vi "Add Record.vi"(8 "error in (no error)":errorcluster, 9 "Channel List":string, 10 "Waveforms":T1(array[cluster]), 11 "Live Graph Plotter in":refnum<class "Live Graph Plotter.lvclass">) -> (0 "error out":errorcluster, 3 "Live Graph Plotter out":refnum<class "Live Graph Plotter.lvclass">)   [LabVIEW 2025, in "Live Graph Plotter.lvclass"]
uses:
  Live Graph Plotter.lvclass
  Live Graph Plotter.lvclass/Live Graph Plotter.ctl
  <vilib>/ErrorRing/Error Ring.xnode
  <vilib>/Utility/error.llb/Error Cluster From Error Code.vi
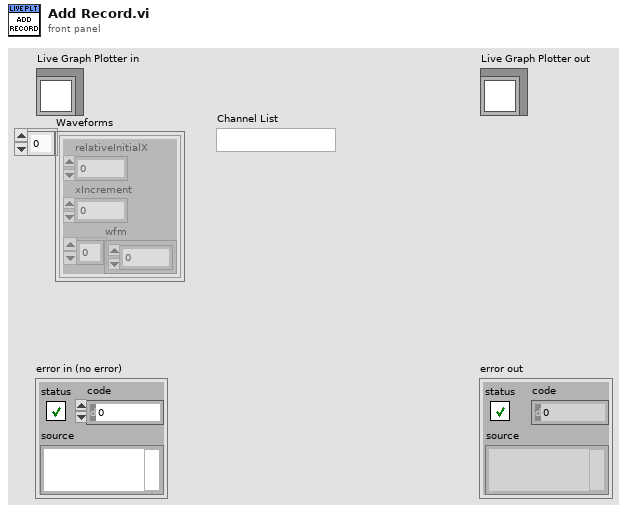
[diagram p1: front panel]
types:
  T1 = cluster{"relativeInitialX":dbl, "xIncrement":dbl, "wfm":dbl[]}[]
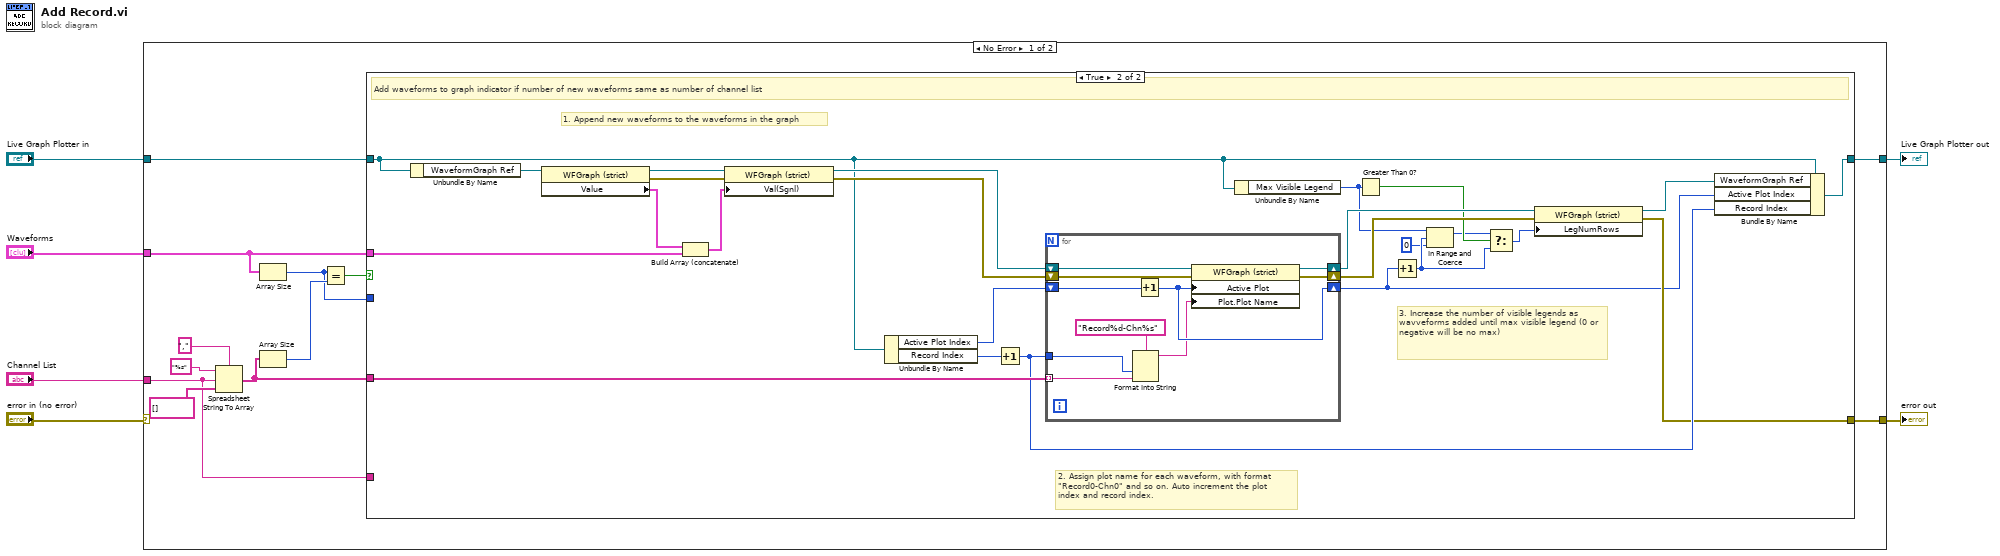
[diagram p0: block diagram]
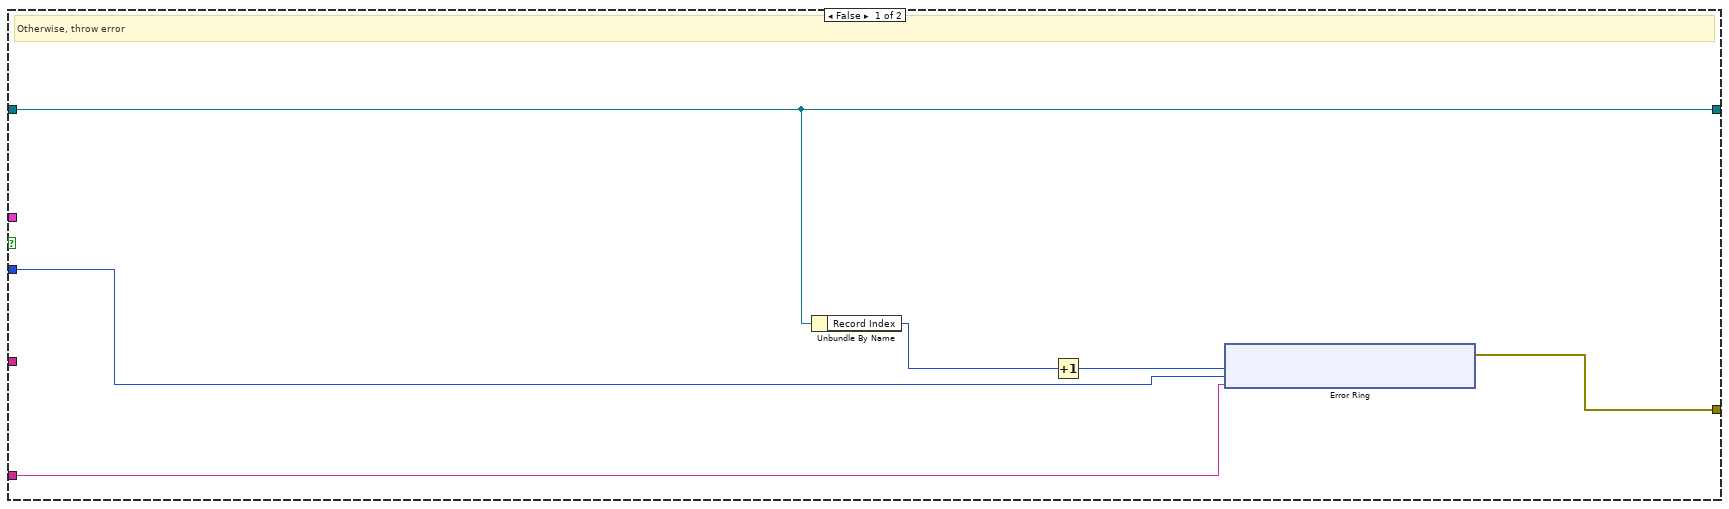
[diagram p2: hidden frame]
diagram:
  n1 = case shown="No Error" "error in (no error)" {
    selector: "error in (no error)" -> [_ w70]
    tunnel: [w10 w70] -> w5
    tunnel: [w18 w69] -> w3
    tunnel: "Live Graph Plotter in" -> [w11 w69]
    tunnel: "Waveforms" -> [w14 _]
    tunnel: "Channel List" -> [w7 _]
    frame No Error {
      n2 = Spreadsheet String To Array(delimiter (Tab)=",", format string="%s", spreadsheet string=w7, array type (2D Dbl)=string[] []) -> (array=w12:string[])
      n3 = Array Size(array=w14) -> (size(s)=w8:i32)
      n4 = Array Size(array=w12) -> (size(s)=w13:i32)
      n5 = Equal?(x=w8, y=w13) -> (x = y?=w9:bool)
      n6 = case shown="True" w9 {
        tunnel: [w24 w58] -> w18
        tunnel: w14 -> [_ w54]
        tunnel: w12 -> [_ w53]
        tunnel: w11 -> [w24 w40]
        tunnel: [w19 w45] -> w10
        tunnel: w8 -> [w21 _]
        tunnel: w7 -> [w20 _]
        frame False {
          # "Otherwise, throw error"
          n7 = Unbundle By Name(w24) -> ("Record Index"=w23:i32)
          n8 = Increment(x=w23) -> (x+1=w22:i32)
          n9 = xnode "Error Ring"("parameter 0"=w22, "parameter 1"=w21, "parameter 2"=w20) -> ("error out"=w19:errorcluster)
        }
        frame True {
          # "3. Increase the number of visible legends as wavveforms added until max visible legend (0 or negative will be no max)"
          # "2. Assign plot name for each waveform, with format\n\"Record0-Chn0\" and so on. Auto increment the plot\nindex and record index."
          # "1. Append new waveforms to the waveforms in the graph"
          # "Add waveforms to graph indicator if number of new waveforms same as number of channel list"
          n10 = Unbundle By Name(w40) -> ("WaveformGraph Ref"=w41:refnum<vi>)
          n11 = property class="WFGraph (strict)"(reference=w41) -> (reference out=w57:refnum<vi>, error out=w56:errorcluster, "Value"=w55:T1)  [unwired: 1 in]
          n12 = Build Array (concatenate)(w55, w54) -> (w46:T1)
          n13 = property class="WFGraph (strict)"(reference=w57, error in=w56, "Val(Sgnl)"=w46) -> (reference out=w52:refnum<vi>, error out=w51:errorcluster)
          n14 = Unbundle By Name(w40) -> ("Active Plot Index"=w49:i32, "Record Index"=w50:i32)
          n15 = Increment(x=w50) -> (x+1=w48:i32)
          n16 = for {
            tunnel: w53 -> [w67] mode=indexing
            tunnel: w48 -> [w66]
            shift-right: [w65] -> w44
            shift-left: w52 -> [w64]
            shift-right: [w62] -> w47
            shift-left: w51 -> [w63]
            shift-right: [w60] -> w42
            shift-left: w49 -> [w61]
            n17 = Format Into String(format string="Record%d-Chn%s", w66, w67) -> (resulting string=w59:string)  [unwired: 2 in, 1 out]
            n18 = Increment(x=w61) -> (x+1=w60:i32)
            n19 = property class="WFGraph (strict)"(reference=w64, error in=w63, "Active Plot"=w60, "Plot.Plot Name"=w59) -> (reference out=w65:refnum<vi>, error out=w62:errorcluster)
          }
          n20 = Unbundle By Name(w40) -> ("Max Visible Legend"=w36:i32)
          n21 = Greater Than 0?(x=w36) -> (x > 0?=w39:bool)
          n22 = Increment(x=w42) -> (x+1=w37:i32)
          n23 = In Range and Coerce(upper limit=w36, x=w37, lower limit=0) -> (coerced(x)=w34:i32)  [unwired: 1 out]
          n24 = Select(t=w34, s=w39, f=w37) -> (s? t:f=w38:i32)
          n25 = property class="WFGraph (strict)"(reference=w44, error in=w47, "LegNumRows"=w38) -> (reference out=w43:refnum<vi>, error out=w45:errorcluster)
          n26 = Bundle By Name(cluster=w40, "WaveformGraph Ref"=w43, "Active Plot Index"=w42, "Record Index"=w48) -> (w58:refnum<class "Live Graph Plotter.lvclass">)
        }
      }
    }
    frame Error {
    }
  }
  "error out" <- w5
  "Live Graph Plotter out" <- w3
